vi "Test String Subset.vi"(8 "error in (no error)":errorcluster) -> (0 "error out":errorcluster, 3 "Pass?":bool)   [LabVIEW 2020]
uses:
  G-Unicode/Types/UTF-8 String/UTF-8 String.lvclass/UTF-8 String.ctl
  6c3bdbaa-dd8a-4d7a-a6b3-47bb84b7ab58.vi
  264a07c0-f4c2-4ea3-88ef-a13d84b4d497.vi
  45aec575-2979-4ee1-8716-e0589e8f3a80.vi
  310073a2-a64f-4bb1-b41b-518da9507cbb.vi
  52367a98-e987-492e-8e34-06f004b52f76.vi
  0032c660-e719-47bc-bfae-3eb3c0e15da0.vi
  908b0875-7fce-4a01-b2dd-ed181c2719e3.vi
  e45cf646-96a9-420e-b517-089b6751d525.vi
  G-Unicode/Private/Conversion/String as Encoded String.vi
  G-Unicode/Private/Conversion/Polymorphic VIs/String as Encoded String (UTF-8 String).vi
  G-Unicode/Private/Library/gu_string_subset.vi
  264a07c0-f4c2-4ea3-88ef-a13d84b4d497.vi/3a31b270-3bb6-4c58-a256-c5fcc2c98f09.vi
  264a07c0-f4c2-4ea3-88ef-a13d84b4d497.vi/0ec5df2d-ef9b-4f84-a6a8-ffcedd45c4dc.vi
  310073a2-a64f-4bb1-b41b-518da9507cbb.vi/3a31b270-3bb6-4c58-a256-c5fcc2c98f09.vi
  310073a2-a64f-4bb1-b41b-518da9507cbb.vi/0ec5df2d-ef9b-4f84-a6a8-ffcedd45c4dc.vi
  G-Unicode/Private/Conversion/Polymorphic VIs/String as Encoded String (LabVIEW String).vi
  0032c660-e719-47bc-bfae-3eb3c0e15da0.vi/3a31b270-3bb6-4c58-a256-c5fcc2c98f09.vi
  0032c660-e719-47bc-bfae-3eb3c0e15da0.vi/0ec5df2d-ef9b-4f84-a6a8-ffcedd45c4dc.vi
  e45cf646-96a9-420e-b517-089b6751d525.vi/3a31b270-3bb6-4c58-a256-c5fcc2c98f09.vi
  e45cf646-96a9-420e-b517-089b6751d525.vi/0ec5df2d-ef9b-4f84-a6a8-ffcedd45c4dc.vi
  G-Unicode/Types/UTF-8 String/Read Encoded UTF-8 String.vi
  G-Unicode/Private/Memory/Copy String.vi
  G-Unicode/Private/Library/Result To Error.vi
  G-Unicode/Private/Conversion/Text as Encoded String.vi
  G-Unicode/Private/Conversion/Polymorphic VIs/Text as Encoded String (UTF-8 String).vi
  G-Unicode/Private/Conversion/Text to UTF-8.vi
  G-Unicode/Private/Conversion/Polymorphic VIs/Text to UTF-8 (LabVIEW String).vi
  G-Unicode/Private/Conversion/Polymorphic VIs/Text as Encoded String (LabVIEW String).vi
  G-Unicode/Private/Memory/Copy String.vi/4d47babd-4a2d-4eb7-b91b-7e707d692665.vi
  G-Unicode/Private/Library/gu_free.vi
  <vilib>/Utility/error.llb/Error Cluster From Error Code.vi
  G-Unicode/Types/UTF-8 String/UTF-8 String.lvclass
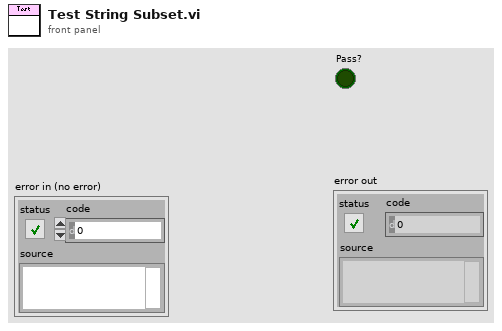
[diagram p1: front panel]
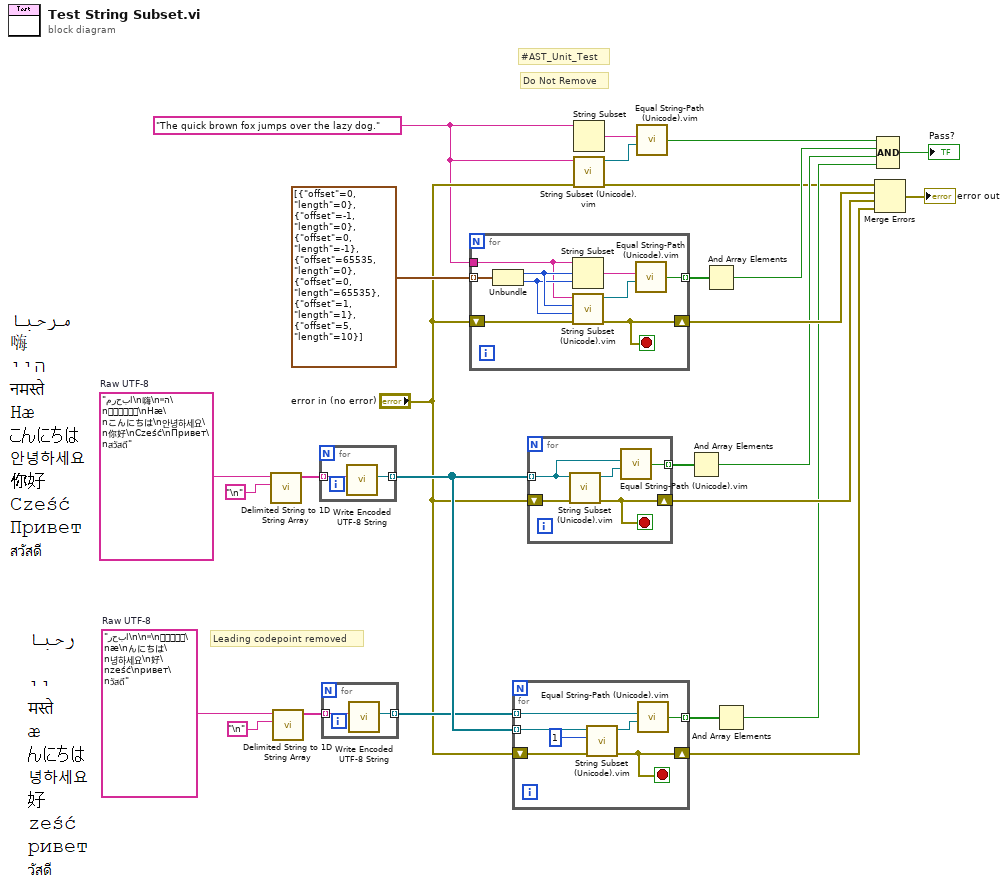
[diagram p0: block diagram]
diagram:
  w10 = "رحبا\n\nיי\nमस्ते\næ\nんにちは\n녕하세요\n好\nześć\nривет\nวัสดี"  # Raw UTF-8
  w1 = "The quick brown fox jumps over the lazy dog." ("string")
  w25 = "مرحبا\n嗨\nהיי\nनमस्ते\nHæ\nこんにちは\n안녕하세요\n你好\nCześć\nПривет\nสวัสดี"  # Raw UTF-8
  # "Leading codepoint removed"
  # "Do Not Remove"
  # "#AST_Unit_Test"
  n1 = call <vilib>:"Delimited String to 1D String Array.vi"("delimiter"="\n", "delimited string"=w25) -> ("string array"=w24:string[])  [unwired: 9 in]
  n2 = call <vilib>:"Delimited String to 1D String Array.vi"("delimiter"="\n", "delimited string"=w10) -> ("string array"=w11:string[])  [unwired: 9 in]
  n3 = for {
    tunnel: w24 -> [w28] mode=indexing
    tunnel: [w27] -> w12 mode=indexing
    n4 = call "Write Encoded UTF-8 String.vi"("Encoded UTF-8 String"=w28) -> ("UTF-8 String"=w27:refnum<class "UTF-8 String.lvclass">)  [unwired: 10 in]
  }
  n5 = for {
    tunnel: w11 -> [w30] mode=indexing
    tunnel: [w29] -> w8 mode=indexing
    n6 = call "Write Encoded UTF-8 String.vi"("Encoded UTF-8 String"=w30) -> ("UTF-8 String"=w29:refnum<class "UTF-8 String.lvclass">)  [unwired: 10 in]
  }
  n7 = for {
    tunnel: [w37] -> w17 mode=indexing
    shift-right: [w38] -> w23
    shift-left: "error in (no error)" -> [w39]
    tunnel: w1 -> [w31]
    tunnel: cluster{"offset":i32, "length":i32}[] [{"offset"=0, "length"=0}, {"offset"=-1, "length"=0}, {"offset"=0, "length"=-1}, {"offset"=65535, "length"=0}, {"offset"=0, "length"=65535}, {"offset"=1, "length"=1}, {"offset"=5, "length"=10}] -> [w35] mode=indexing
    stop <- w38 stop-if-true
    n8 = Unbundle(w35) -> ("offset"=w34:i32, "length"=w33:i32)
    n9 = String Subset(string=w31, offset (0)=w34, length (rest)=w33) -> (substring=w32:string)
    n10 = call "String Subset (Unicode).vim"("error in"=w39, "Length (rest)"=w33, "Offset (0)"=w34, "String"=w31) -> ("error out"=w38:errorcluster, "Substring"=w36:refnum<class "UTF-8 String.lvclass">)  [unwired: 6 in]
    n11 = call "Equal String-Path (Unicode).vim"("y"=w36, "x"=w32) -> ("Equal?"=w37:bool)  [unwired: 7 in, 1 out]
  }
  n12 = for {
    tunnel: w12 -> [w45] mode=indexing
    tunnel: [w44] -> w6 mode=indexing
    shift-right: [w43] -> w4
    shift-left: "error in (no error)" -> [w42]
    tunnel: w8 -> [w40] mode=indexing
    stop <- w43 stop-if-true
    n13 = call "String Subset (Unicode).vim"("error in"=w42, "Offset (0)"=1, "String"=w45) -> ("error out"=w43:errorcluster, "Substring"=w46:refnum<class "UTF-8 String.lvclass">)  [unwired: 7 in]
    n14 = call "Equal String-Path (Unicode).vim"("y"=w46, "x"=w40) -> ("Equal?"=w44:bool)  [unwired: 7 in, 1 out]
  }
  n15 = for {
    tunnel: w12 -> [w47] mode=indexing
    tunnel: [w50] -> w15 mode=indexing
    shift-right: [w49] -> w13
    shift-left: "error in (no error)" -> [w48]
    stop <- w49 stop-if-true
    n16 = call "String Subset (Unicode).vim"("error in"=w48, "String"=w47) -> ("error out"=w49:errorcluster, "Substring"=w51:refnum<class "UTF-8 String.lvclass">)  [unwired: 8 in]
    n17 = call "Equal String-Path (Unicode).vim"("y"=w51, "x"=w47) -> ("Equal?"=w50:bool)  [unwired: 7 in, 1 out]
  }
  n18 = String Subset(string=w1) -> (substring=w3:string)  [unwired: 2 in]
  n19 = call "String Subset (Unicode).vim"("error in"="error in (no error)", "String"=w1) -> ("error out"=w2:errorcluster, "Substring"=w21:refnum<class "UTF-8 String.lvclass">)  [unwired: 8 in]
  n20 = call "Equal String-Path (Unicode).vim"("y"=w21, "x"=w3) -> ("Equal?"=w20:bool)  [unwired: 7 in, 1 out]
  n21 = And Array Elements(Boolean array=w15) -> (logical AND=w14:bool)
  n22 = And Array Elements(Boolean array=w17) -> (logical AND=w16:bool)
  n23 = And Array Elements(Boolean array=w6) -> (logical AND=w5:bool)
  n24 = Merge Errors(w2, w23, w13, w4) -> (→"error out":errorcluster)
  n25 = Compound Arithmetic op=AND(w20, w16, w14, w5) -> (→"Pass?":bool)
